vi "destroy.vi"(8 "error in (no error)":errorcluster, 11 "PositionSignals in":refnum<class "PositionSignals.lvclass">) -> (0 "error out":errorcluster, 3 "PositionSignals out":refnum<class "PositionSignals.lvclass">)   [LabVIEW 2010, in "PositionSignals.lvclass"]
uses:
  PositionSignals.lvclass
  common/classes/ImageCollection/ImageCollection/ImageCollection.lvclass
  PositionSignals.lvclass/PositionSignals.ctl
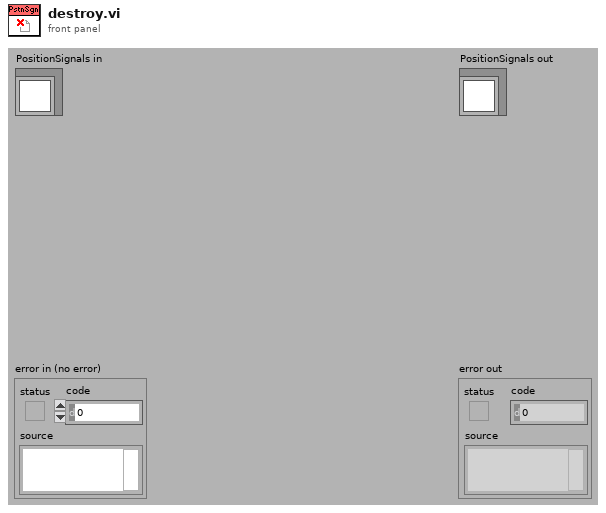
[diagram p1: front panel]
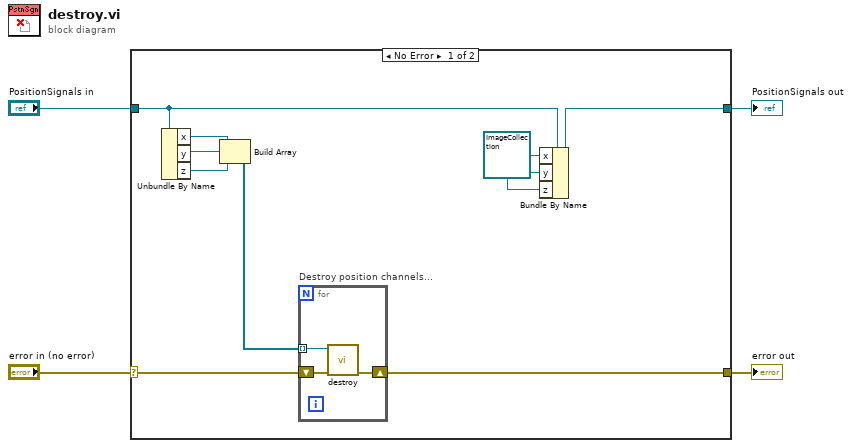
[diagram p0: block diagram]
diagram:
  n1 = case shown="No Error" "error in (no error)" {
    selector: "error in (no error)" -> [w13 w18]
    tunnel: [w12 w18] -> w3
    tunnel: [w5 w17] -> w1
    tunnel: "PositionSignals in" -> [w6 w17]
    frame No Error {
      w7 = refnum<class "ImageCollection.lvclass"> refnum ("x")
      n2 = Unbundle By Name(w6) -> ("x"=w9:refnum<class "ImageCollection.lvclass">, "y"=w10:refnum<class "ImageCollection.lvclass">, "z"=w11:refnum<class "ImageCollection.lvclass">)
      n3 = Build Array(w9, w10, w11) -> (w8:refnum<class "ImageCollection.lvclass">[])
      n4 = for "Destroy position channels..." {
        tunnel: w8 -> [w14] mode=indexing
        shift-right: [w15] -> w12
        shift-left: w13 -> [w16]
        n5 = call-dynamic "destroy.vi"("error in (no error)"=w16, "ImageCollection in"=w14) -> ("error out"=w15:errorcluster)  [unwired: 8 in, 1 out]
      }
      n6 = Bundle By Name(cluster=w6, "x"=w7, "y"=w7, "z"=w7) -> (w5:refnum<class "PositionSignals.lvclass">)
    }
    frame Error {
    }
  }
  "error out" <- w3
  "PositionSignals out" <- w1
